vi "Beam_Max_Pos.vi"(0 "Beam Name":string, 1 "Traverse Name":string, 2 "Fixed Axis only?":bool, 5 "Fixed Axis":T1, 7 "Search Step (mm)":dbl=1.0, 9 "Starting Position":dbl[](array[numeric]) format="%.1f", 11 "Mode":T3, 12 "Wavelength  nm":sgl=533.0 caption="Wavelength (0.0)", 14 "Picture Log":path) -> (3 "Message":string, 4 "Beam maxima":dbl[](array[numeric]) format="%.1f", 10 "Status":T2, 15 "Power at Maxima":dbl)   [LabVIEW 2020]
uses:
  Controls/User_Specific_mode.ctl
  Gen Trav/Multi_Run_Status.ctl
  Controls/Fixed Axis.ctl
  Gen Trav/Trav_mode.ctl
  Controls/Tunnel_Coordinates.ctl
panel:
  out "vi reference":refnum<vi>
  in  "stop":bool
  out "Y":i32
  out "X":i32
  out "Array 2":dbl[](array[numeric]) format="%.4f"
  out "Measured Points":dbl[][](array[numeric]) format="%.2f"
  out "Current Value":dbl format="%.2f"
  out "Current Index":i32
  out "Array":i32[][](array[numeric])
  out "Light Power Measurement":dbl[][](graph)
  out "Found Maxima?":bool
  out "Present Position":dbl[](array[numeric])
  out "Profile":dbl[][](array[numeric]) format="%.2f"
  out "Log File":path
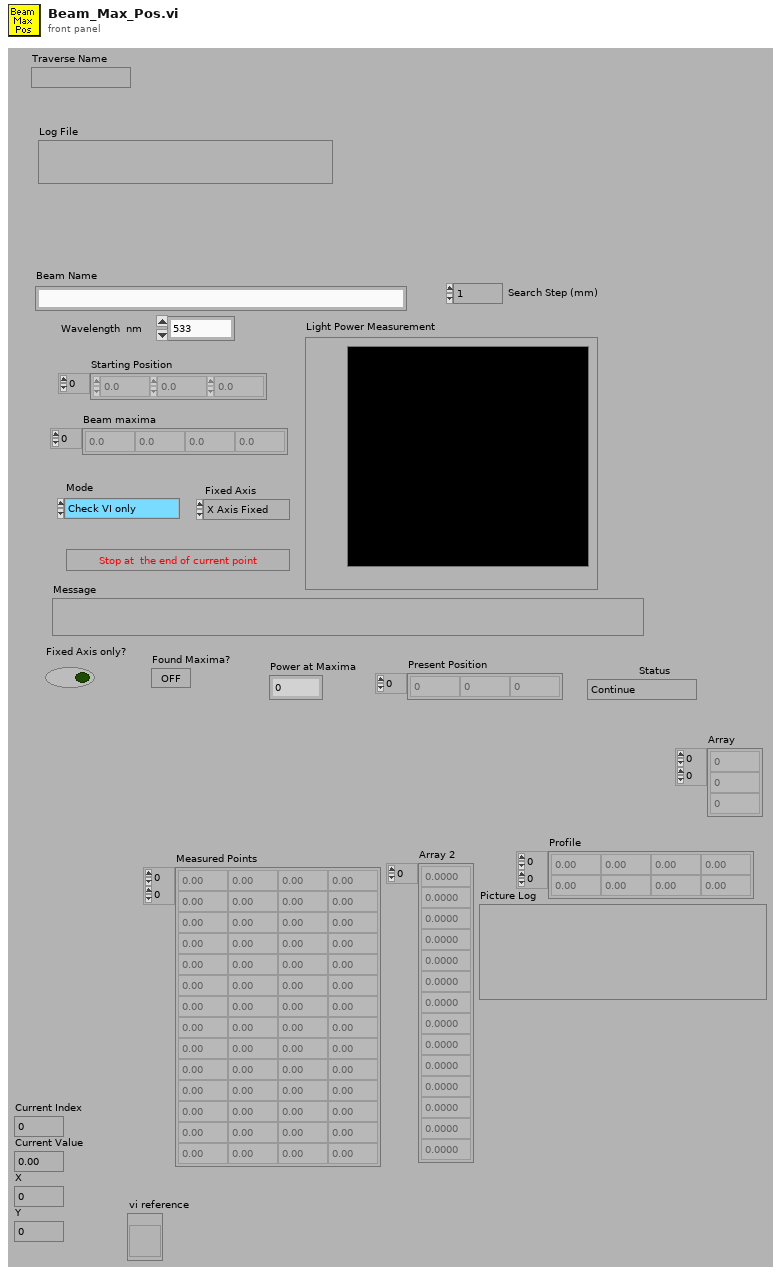
[diagram p1: front panel]
types:
  T1 = typedef "Fixed Axis.ctl" = enum16{"X Axis Fixed", "Y Axis Fixed", "Z Axis Fixed"}
  T2 = typedef "Multi_Run_Status.ctl" = enum16{"Continue", "Continue with Error", "Jump to Next Point", "Jump to Next Row", "Jump To Fall Back", "Terminate Run"}
  T3 = typedef "User_Specific_mode.ctl" = enum16{"Check VI only", "Run VI"}
  T4 = typedef "Tunnel_Coordinates.ctl" = enum16{"Work in Tunnel Coordinates", "Work in Model Coordinates"}
  T5 = typedef "Trav_mode.ctl" = enum16{"Move traverse", "Read traverse position", "Teach Position"}
  T6 = cluster{"second":i32, "minute":i32, "hour":i32, "day of month":i32, "month":i32, "year":i32, "day of week":i32, "day of year":i32, "is DST":i32}
  T7 = typedef "LVRectTypeDef.ctl" = cluster{"left":i16, "top":i16, "right":i16, "bottom":i16}
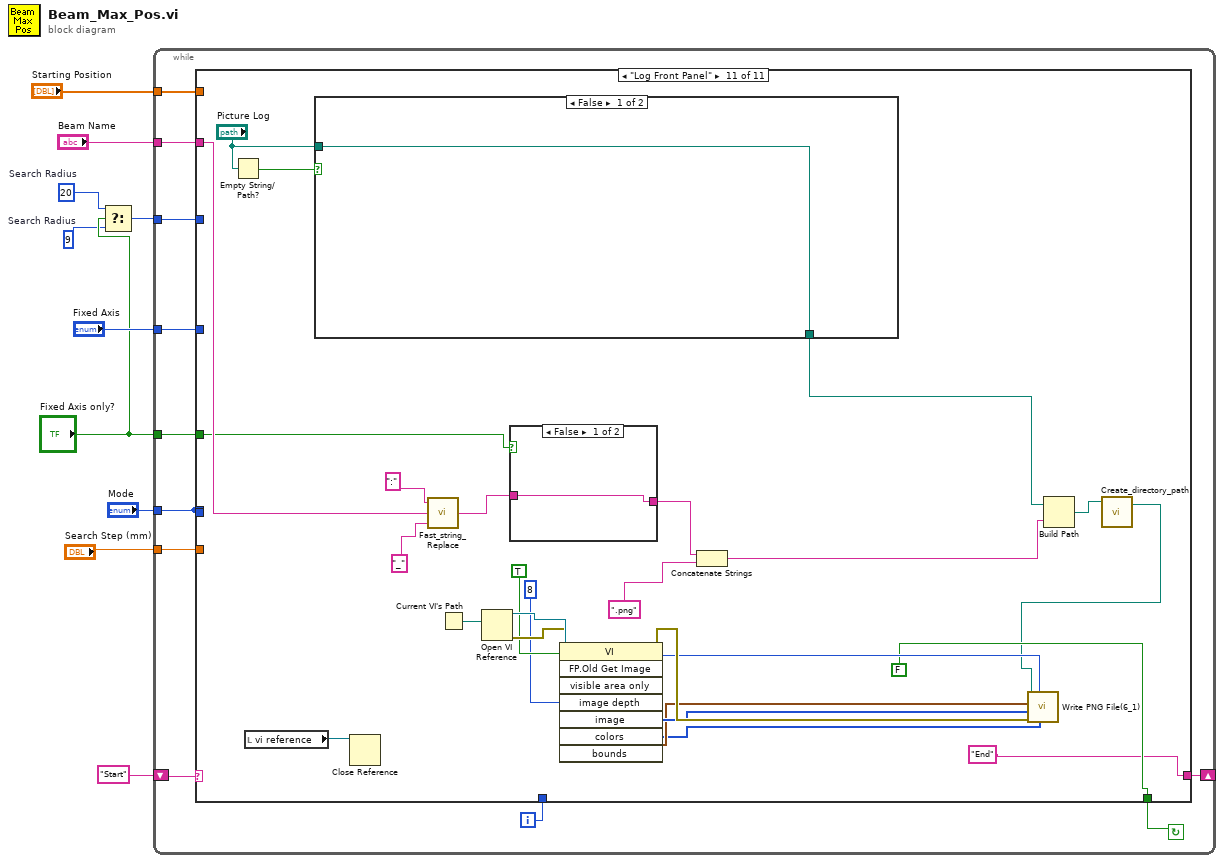
[diagram p0: block diagram]
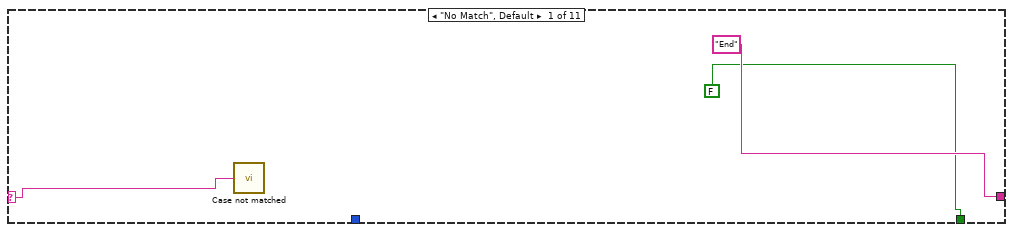
[diagram p2: hidden frame]
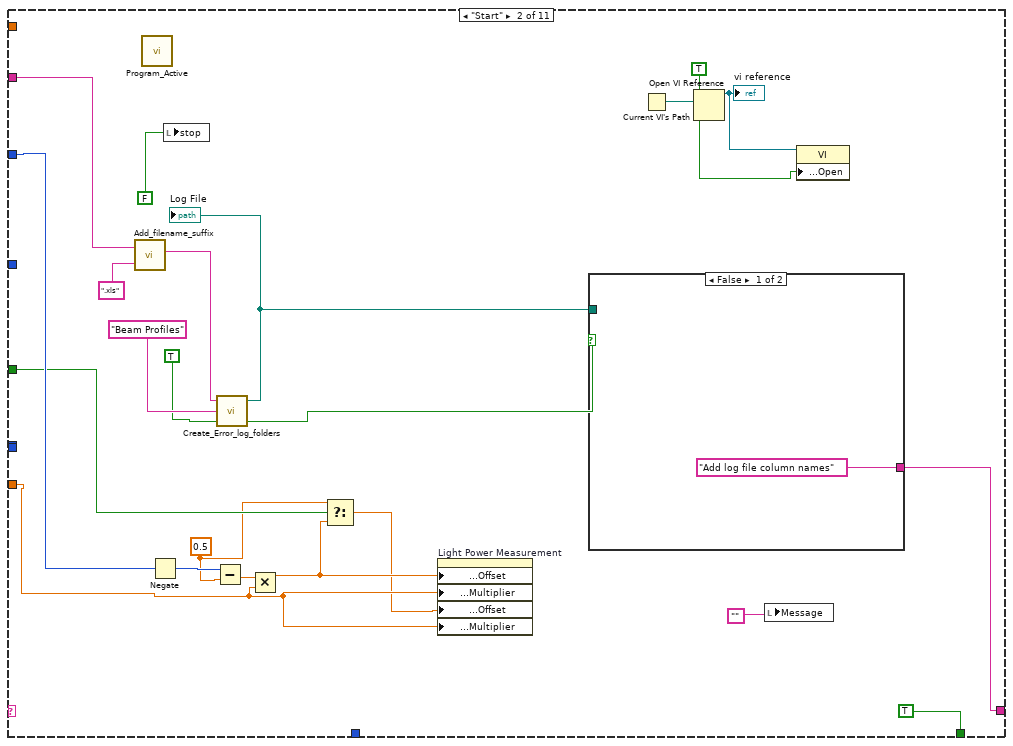
[diagram p3: hidden frame]
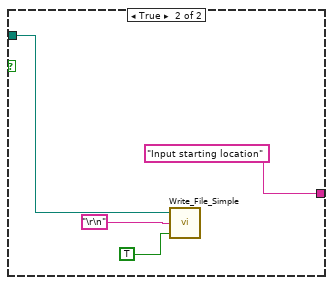
[diagram p4: hidden frame]
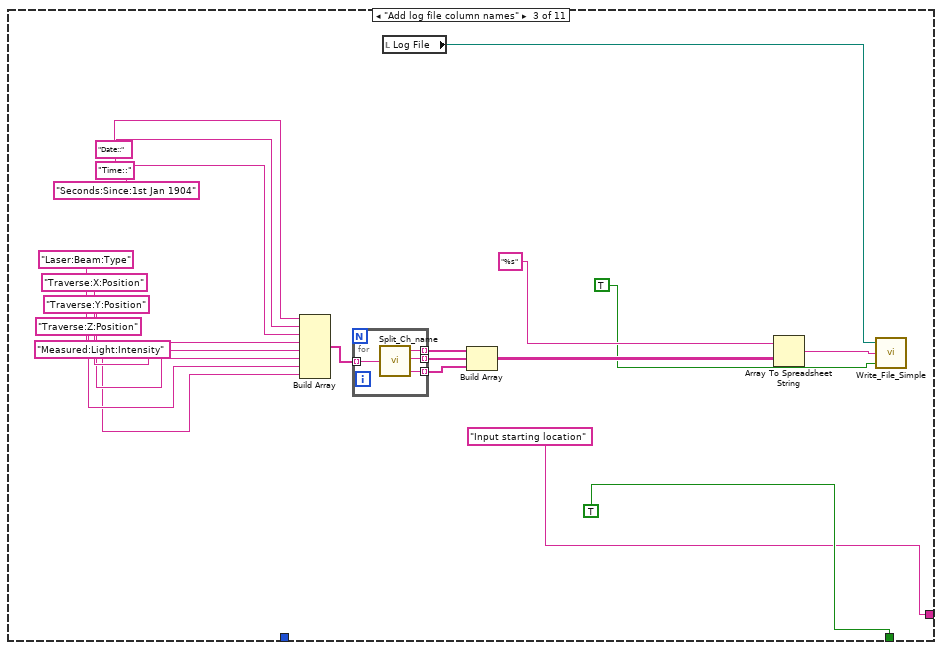
[diagram p5: hidden frame]
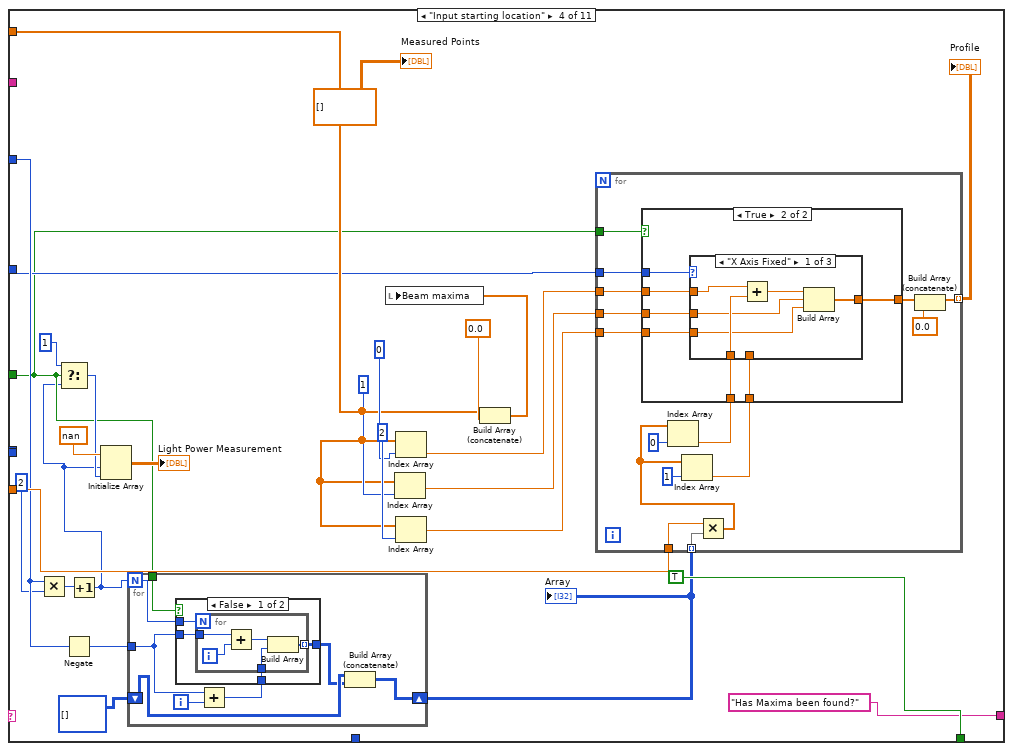
[diagram p6: hidden frame]
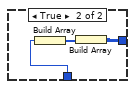
[diagram p7: hidden frame]
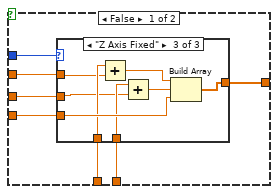
[diagram p8: hidden frame]
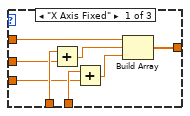
[diagram p9: hidden frame]
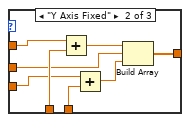
[diagram p10: hidden frame]
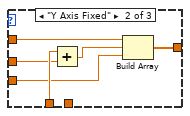
[diagram p11: hidden frame]
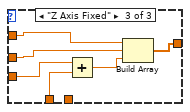
[diagram p12: hidden frame]
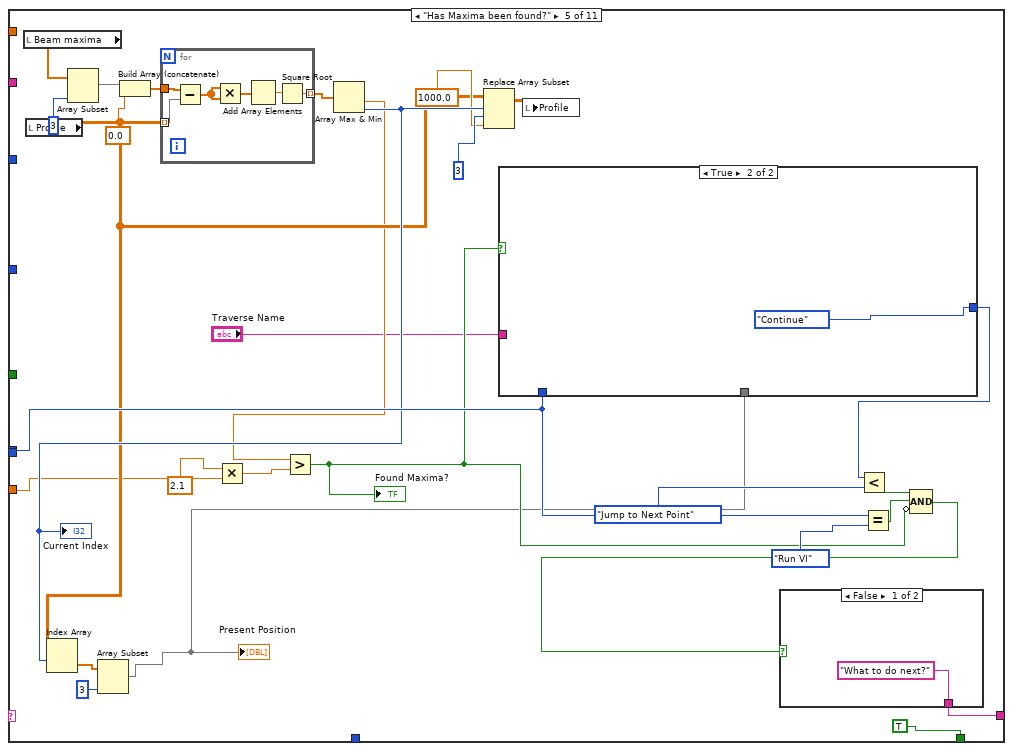
[diagram p13: hidden frame]
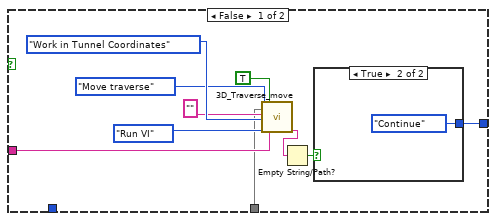
[diagram p14: hidden frame]
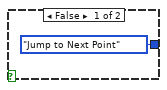
[diagram p15: hidden frame]
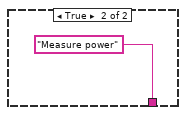
[diagram p16: hidden frame]
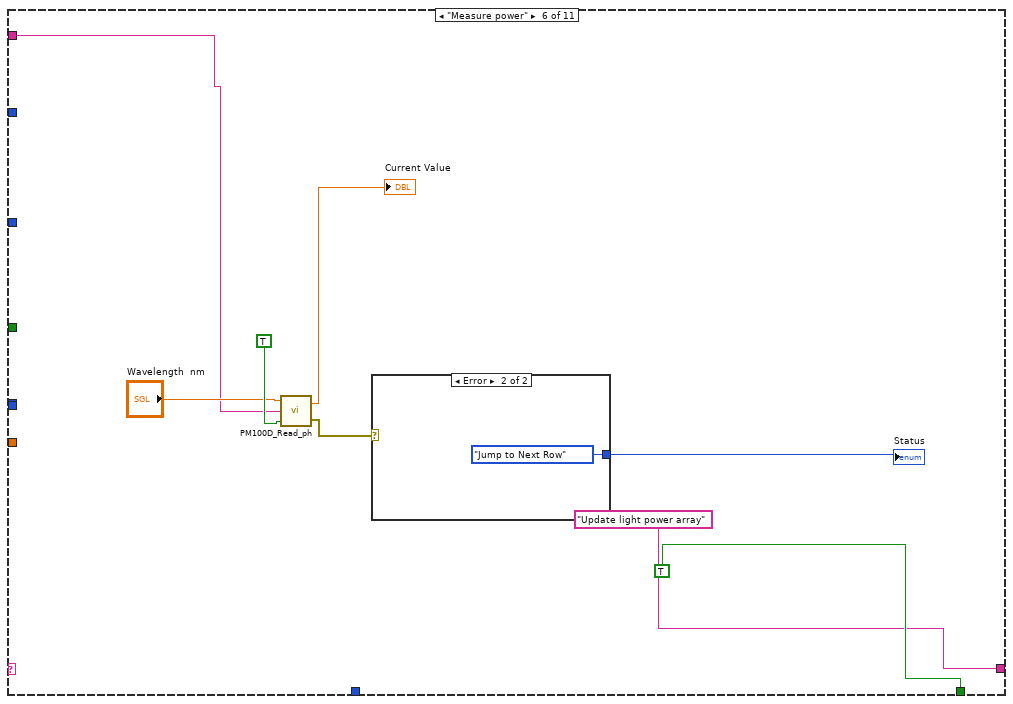
[diagram p17: hidden frame]
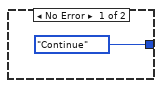
[diagram p18: hidden frame]
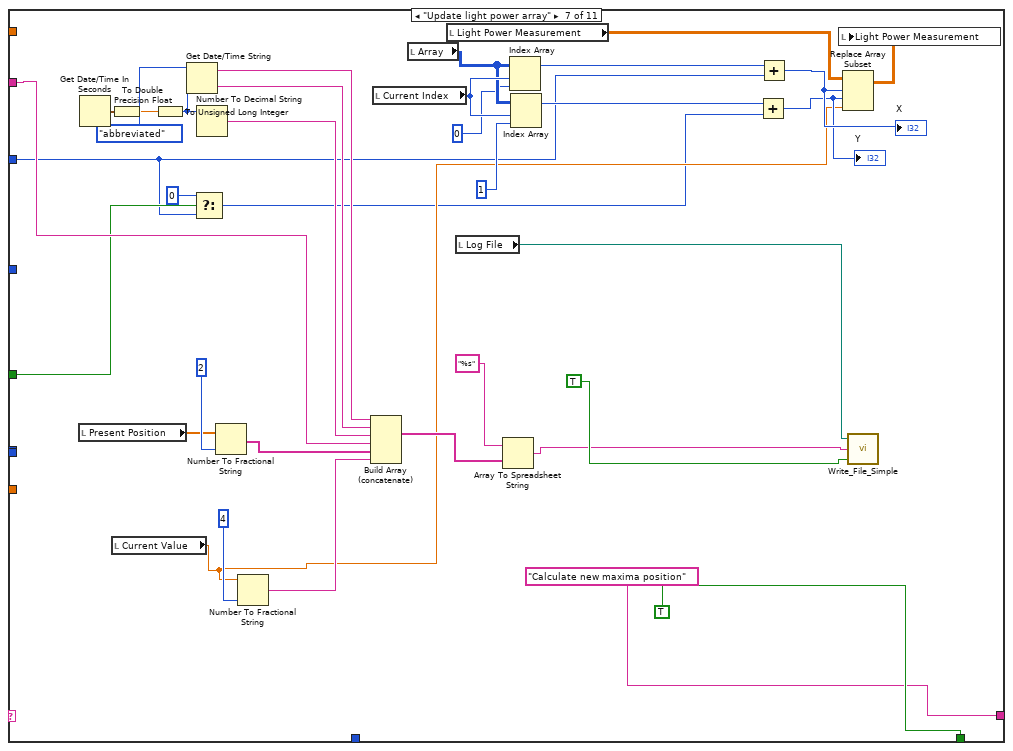
[diagram p19: hidden frame]
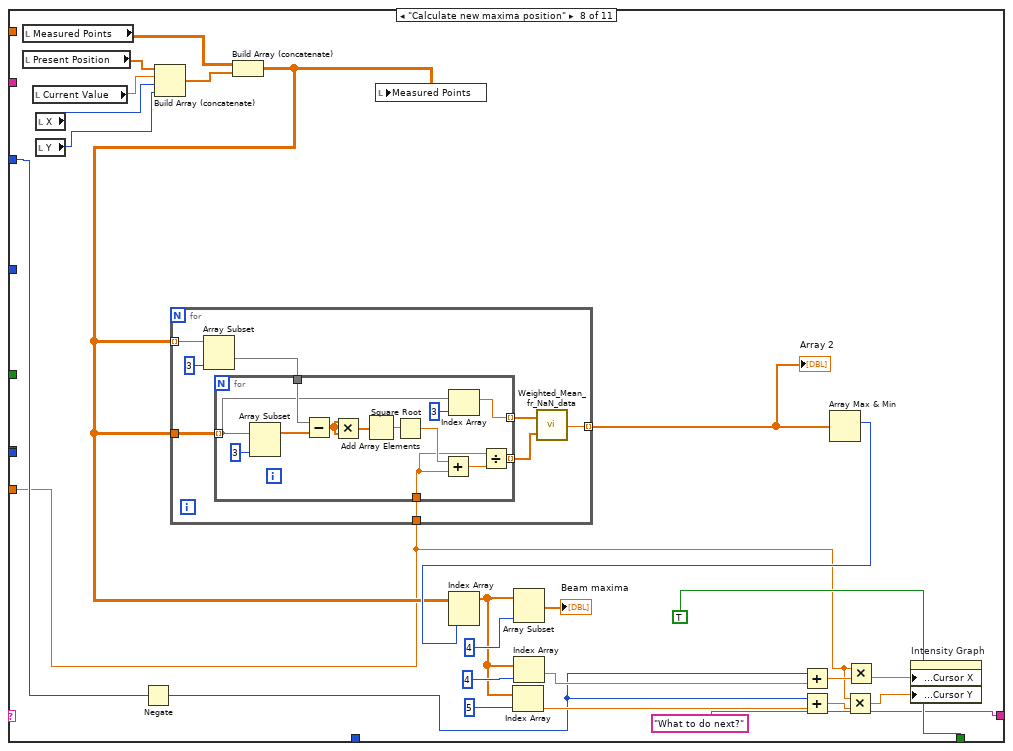
[diagram p20: hidden frame]
diagram:
  w1 = 20  # Search Radius
  w2 = 9  # Search Radius
  n1 = Select(t=w1, s="Fixed Axis only?", f=w2) -> (s? t:f=w4:i32)
  n2 = while {
    tunnel: "Search Step (mm)" -> [w18]
    tunnel: "Mode" -> [w19]
    shift-left: "Start" -> [w13]
    shift-right: [w20] -> _
    tunnel: w4 -> [w17]
    tunnel: "Beam Name" -> [w16]
    tunnel: "Starting Position" -> [w15]
    tunnel: "Fixed Axis" -> [w12]
    tunnel: "Fixed Axis only?" -> [w11]
    i -> [w14]
    stop <- w21 continue-if-true
    n3 = case shown="\"Log Front Panel\"" w13 {
      selector: w13 -> [w22 _ _ _ _ _ _ _ _ _ _]
      tunnel: w19 -> [_ _ _ _ w219 _ _ _ w340 _ _]
      tunnel: [FALSE TRUE TRUE TRUE TRUE TRUE TRUE TRUE w334 TRUE FALSE] -> w21
      tunnel: ["End" w36 "Input starting location" "Has Maxima been found?" w200 "Update light power array" "Calculate new maxima position" "What to do next?" w337 "Log Front Panel" "End"] -> w20
      tunnel: w19 -> [_ _ _ _ _ _ _ _ _ _ _]
      tunnel: w18 -> [_ w31 _ w94 w201 _ _ w291 _ _ _]
      tunnel: w17 -> [_ w41 _ w88 _ _ w255 w295 _ _ _]
      tunnel: w16 -> [_ w39 _ _ _ w243 w261 _ _ w358 w407]
      tunnel: w15 -> [_ _ _ w82 _ _ _ _ _ w357 _]
      tunnel: w14 -> [_ _ _ _ _ _ _ _ _ _ _]
      tunnel: w12 -> [_ _ _ w80 _ _ _ _ _ _ _]
      tunnel: w11 -> [_ w28 _ w76 _ _ w256 _ _ _ w404]
      frame "No Match", Default {
        n4 = call "Case not matched.vi"("Case Name not Matched"=w22) -> ()
      }
      frame "Start" {
        w25 = 0.5 ("y")
        n5 = call "Add_filename_suffix.vi"("Filename"=w39, "Suffix to add"=".xls") -> ("Filename out"=w37:string)  [unwired: 3 out]
        n6 = call "Program_Active.vi"() -> ()  [unwired: 1 in]
        n7 = Negate(x=w41) -> (-x=w29:i32)
        n8 = local write "stop"(FALSE ("stop")) -> ()
        n9 = Subtract(x=w29, y=w25) -> (x-y=w30:dbl)
        n10 = call "Create_Error_log_folders.vi"("Log Filename"=w37, "Log Folder"="Beam Profiles" ("Input Element"), "Per Day Log File?"=TRUE) -> ("Local Log File"=w45:path, "exists?"=w44:bool)  [unwired: 3 in]
        "Log File" <- w45
        n11 = Multiply(x=w30, y=w31) -> (x*y=w27:dbl)
        n12 = Select(t=w25, s=w28, f=w27) -> (s? t:f=w26:dbl)
        n13 = property on="Light Power Measurement" class="IntGraph (strict)"("X Scale.Offset and Multiplier:Offset"=w27, "X Scale.Offset and Multiplier:Multiplier"=w31, "Y Scale.Offset and Multiplier:Offset"=w26, "Y Scale.Offset and Multiplier:Multiplier"=w31) -> ()  [unwired: 2 in, 2 out]
        n14 = case shown="False" w44 {
          tunnel: w45 -> [_ w48]
          tunnel: ["Add log file column names" "Input starting location"] -> w36
          frame False {
          }
          frame True {
            n15 = call "Write_File_Simple.vi"("append to file? (new file:F)"=TRUE, "character string"="\r\n", "file path"=w48) -> ()  [unwired: 2 out]
          }
        }
        n16 = Current VI's Path() -> (path=w35:path)
        n17 = Open VI Reference(vi path=w35) -> (vi reference=w34:refnum<vi>)  [unwired: 1 in, 5 out]
        "vi reference" <- w34
        n18 = local write "Message"("") -> ()
        n19 = property class="VI"(reference=w34, "Front Panel Window:Open"=TRUE) -> ()  [unwired: 1 in, 2 out]
      }
      frame "Add log file column names" {
        n20 = Build Array("Date::", "Time::", "Seconds:Since:1st Jan 1904", "Laser:Beam:Type", "Traverse:X:Position", "Traverse:Y:Position", "Traverse:Z:Position", "Measured:Light:Intensity") -> (w64:string[])
        n21 = for {
          tunnel: w64 -> [w74] mode=indexing
          tunnel: [w73] -> w65 mode=indexing
          tunnel: [w72] -> w66 mode=indexing
          tunnel: [w71] -> w67 mode=indexing
          n22 = call "Split_Ch_name.vi"("Ch name"=w74) -> ("Top level"=w73:string, "Middle"=w72:string, "Low level"=w71:string)
        }
        n23 = local read "Log File"() -> (w52:path)
        n24 = Build Array(w65, w66, w67) -> (w62:string[][])
        n25 = Array To Spreadsheet String(array=w62, 3:"%s" ("format string")) -> (spreadsheet string=w53:string)  [unwired: 1 out]
        n26 = call "Write_File_Simple.vi"("append to file? (new file:F)"=TRUE, "character string"=w53, "file path"=w52) -> ()  [unwired: 2 out]
      }
      frame "Input starting location" {
        n27 = Multiply(x=w88, y=2) -> (x*y=w86:i32)
        n28 = Negate(x=w88) -> (-x=w77:i32)
        n29 = Increment(x=w86) -> (x+1=w75:i32)
        n30 = Select(t=1, s=w76, f=w75) -> (s? t:f=w78:i32)
        n31 = Initialize Array(nan, w75, w78) -> (→"Light Power Measurement":dbl[][])
        n32 = for {
          N: w75 -> [w102]
          tunnel: w77 -> [w103]
          shift-right: [w105] -> w92
          shift-left: i32[][] [] -> [w107]
          tunnel: w76 -> [w104]
          i -> [w109]
          n33 = Add(x=w103, y=w109) -> (x+y=w108:i32)
          n34 = case shown="False" w104 {
            tunnel: w108 -> [w113 w120]
            tunnel: [w112 w121] -> w106
            tunnel: w103 -> [w111 _]
            tunnel: w102 -> [w110 _]
            frame False {
              n35 = for {
                N: w110 -> [_]
                tunnel: w111 -> [w117]
                tunnel: w113 -> [w115]
                tunnel: [w114] -> w112 mode=indexing
                i -> [w118]
                n36 = Add(x=w117, y=w118) -> (x+y=w116:i32)
                n37 = Build Array(w116, w115) -> (w114:i32[])
              }
            }
            frame True {
              n38 = Build Array(w120) -> (w119:i32[])
              n39 = Build Array(w119) -> (w121:i32[][])
            }
          }
          n40 = Build Array (concatenate)(w107, w106) -> (w105:i32[][])
        }
        "Array" <- w92
        n41 = Index Array(array=w82, index=1 ("Index")) -> (element=w98:dbl)
        n42 = Index Array(array=w82, index=0 ("Index")) -> (element=w99:dbl)
        n43 = Index Array(array=w82, index=2 ("Index")) -> (element=w97:dbl)
        n44 = Build Array (concatenate)(w82, 0.0 ("Numeric")) -> (w95:dbl[])
        n45 = local write "Beam maxima"(w95) -> ()
        n46 = for {
          tunnel: w94 -> [w136]
          tunnel: w92 -> [w135] mode=indexing
          tunnel: w80 -> [w134]
          tunnel: w99 -> [w130]
          tunnel: w98 -> [w127]
          tunnel: w97 -> [w126]
          tunnel: [w124] -> w100 mode=indexing
          tunnel: w76 -> [w122]
          n47 = Multiply(x=w136, y=w135) -> (x*y=w131:dbl[])
          n48 = Index Array(array=w131, index=0 ("Index")) -> (element=w129:dbl)
          n49 = Index Array(array=w131, index=1 ("Index")) -> (element=w128:dbl)
          n50 = case shown="True" w122 {
            tunnel: w134 -> [w143 w174]
            tunnel: w130 -> [w142 w173]
            tunnel: w129 -> [w141 w172]
            tunnel: w128 -> [w140 w171]
            tunnel: w127 -> [w139 w170]
            tunnel: w126 -> [w138 w169]
            tunnel: [w137 w168] -> w125
            frame False {
              n51 = case shown="\"Z Axis Fixed\"" w143 {
                tunnel: w142 -> [w151 w158 w162]
                tunnel: w141 -> [w150 w156 w165]
                tunnel: w140 -> [w149 w155 w164]
                tunnel: w139 -> [w148 w152 w163]
                tunnel: w138 -> [w147 w154 w166]
                tunnel: [w144 w159 w167] -> w137
                frame "X Axis Fixed" {
                  n52 = Add(x=w150, y=w148) -> (x+y=w146:dbl)
                  n53 = Add(x=w149, y=w147) -> (x+y=w145:dbl)
                  n54 = Build Array(w151, w146, w145) -> (w144:dbl[])
                }
                frame "Y Axis Fixed" {
                  n55 = Add(x=w158, y=w156) -> (x+y=w157:dbl)
                  n56 = Add(x=w154, y=w155) -> (x+y=w153:dbl)
                  n57 = Build Array(w157, w152, w153) -> (w159:dbl[])
                }
                frame "Z Axis Fixed" {
                  n58 = Add(x=w165, y=w162) -> (x+y=w161:dbl)
                  n59 = Add(x=w164, y=w163) -> (x+y=w160:dbl)
                  n60 = Build Array(w161, w160, w166) -> (w167:dbl[])
                }
              }
            }
            frame True {
              n61 = case shown="\"X Axis Fixed\"" w174 {
                tunnel: w173 -> [w179 w186 w191]
                tunnel: w172 -> [w177 w185 w188]
                tunnel: w171 -> [_ _ _]
                tunnel: w170 -> [w176 w184 w190]
                tunnel: w169 -> [w175 w181 w189]
                tunnel: [w180 w182 w192] -> w168
                frame "X Axis Fixed" {
                  n62 = Add(x=w179, y=w177) -> (x+y=w178:dbl)
                  n63 = Build Array(w178, w176, w175) -> (w180:dbl[])
                }
                frame "Y Axis Fixed" {
                  n64 = Add(x=w185, y=w184) -> (x+y=w183:dbl)
                  n65 = Build Array(w186, w183, w181) -> (w182:dbl[])
                }
                frame "Z Axis Fixed" {
                  n66 = Add(x=w189, y=w188) -> (x+y=w187:dbl)
                  n67 = Build Array(w191, w190, w187) -> (w192:dbl[])
                }
              }
            }
          }
          n68 = Build Array (concatenate)(w125, 0.0 ("Input Element")) -> (w124:dbl[])
        }
        "Profile" <- w100
        "Measured Points" <- dbl[][] [] ("Measured Points")
      }
      frame "Has Maxima been found?" {
        n69 = local read "Beam maxima"() -> (w217:dbl[])
        n70 = local read "Profile"() -> (w207:dbl[][])
        n71 = Array Subset(array=w217, length=3 ("Array Length")) -> (w214:dbl[])  [unwired: 1 in]
        n72 = Build Array (concatenate)(w214, 0.0 ("Input Element")) -> (w213:dbl[])
        n73 = for {
          tunnel: w207 -> [w242] mode=indexing
          tunnel: w213 -> [w241]
          tunnel: [w237] -> w215 mode=indexing
          n74 = Subtract(x=w241, y=w242) -> (x-y=w239:dbl[])
          n75 = Multiply(x=w239, y=w239) -> (x*y=w238:dbl[])
          n76 = Add Array Elements(numeric array=w238) -> (sum=w240:dbl)
          n77 = Square Root(x=w240) -> (sqrt(x)=w237:dbl)
        }
        n78 = Multiply(x=2.1, y=w201) -> (x*y=w204:dbl)
        n79 = Array Max & Min(array=w215) -> (min value=w205:dbl, min index (indices)=w211:i32)  [unwired: 2 out]
        "Current Index" <- w211
        n80 = Index Array(array=w207, index (row)=w211) -> (element=w197:dbl[])  [unwired: 1 in]
        n81 = Array Subset(array=w197, length=3) -> (w194:dbl[])  [unwired: 1 in]
        "Present Position" <- w194
        n82 = Greater?(x=w205, y=w204) -> (0:w198:bool)
        "Found Maxima?" <- w198
        n83 = Replace Array Subset(array=w207, new element=1000.0 ("Element Data"), index (row)=w211, index (col)=3 ("Index")) -> (w208:dbl[][])
        n84 = case shown="True" w198 {
          tunnel: w219 -> [_ _]
          tunnel: "Traverse Name" -> [w226 _]
          tunnel: w194 -> [w225 _]
          tunnel: [w222 Multi_Run_Status."Continue" ("Status")] -> w193
          frame False {
            n85 = call "3D_Traverse_move.vi"("Mode"=Trav_mode."Move traverse", "Position"=w225, "Extra command String"="", "Work in Tunnel Coordinates"=Tunnel_Coordinates."Work in Tunnel Coordinates", "Simulate/Run"=User_Specific_mode."Run VI", "Route Checking?"=TRUE, "Traverse name"=w226) -> ("Error String"=w224:string)  [unwired: 9 in, 3 out]
            n86 = Empty String/Path?(string/path=w224) -> (empty?=w223:bool)
            n87 = case shown="True" w223 {
              tunnel: [Multi_Run_Status."Jump to Next Point" ("Status") Multi_Run_Status."Continue" ("Status")] -> w222
              frame False {
              }
              frame True {
              }
            }
          }
          frame True {
          }
        }
        n88 = local write "Profile"(w208) -> ()
        n89 = Less?(x=w193, y=Multi_Run_Status."Jump to Next Point" ("Status")) -> (x < y?=w203:bool)
        n90 = Equal?(x=w219, y=User_Specific_mode."Run VI" ("Mode")) -> (x = y?=w202:bool)
        n91 = Compound Arithmetic op=AND(w203, w202, invert w198) -> (w199:bool)
        n92 = case shown="False" w199 {
          tunnel: ["What to do next?" "Measure power"] -> w200
          frame False {
          }
          frame True {
          }
        }
      }
      frame "Measure power" {
        n93 = call "PM100D_Read_ph.vi"("stop"=TRUE, "Beam Name"=w243, "Wavelength (0.0)"="Wavelength  nm") -> ("error out"=w245:errorcluster, "Average Power (mW)"=→"Current Value":dbl)
        n94 = case shown="Error" w245 {
          tunnel: [Multi_Run_Status."Continue" ("Status") Multi_Run_Status."Jump to Next Row" ("Status")] -> w244
          frame No Error {
          }
          frame Error {
          }
        }
        "Status" <- w244
      }
      frame "Update light power array" {
        n95 = local read "Present Position"() -> (w274:dbl[])
        n96 = Get Date/Time In Seconds() -> (seconds since 1Jan1904=w263:timestamp)
        n97 = To Double Precision Float(number=w263) -> (double precision float=w284:dbl)
        n98 = local read "Current Value"() -> (w257:dbl)
        n99 = To Unsigned Long Integer(number=w284) -> (unsigned 32bit integer=w283:u32)
        n100 = Get Date/Time String(date format (0)=enum16{"short", "long", "abbreviated"}."abbreviated", seconds (now)=w283) -> (date string=w282:string, time string=w281:string)  [unwired: 1 out]
        n101 = Select(t=0, s=w256, f=w255) -> (s? t:f=w253:i32)
        n102 = Number To Decimal String(number=w283) -> (decimal integer string=w280:string)  [unwired: 1 out]
        n103 = Number To Fractional String(number=w274, precision (6)=i16 2) -> (F-format string=w275:string[])  [unwired: 2 out]
        n104 = Number To Fractional String(number=w257, precision (6)=i16 4) -> (F-format string=w276:string)  [unwired: 2 out]
        n105 = Build Array (concatenate)(w282, w281, w280, w261, w275, w276) -> (w279:string[])
        n106 = local read "Current Index"() -> (w273:i32)
        n107 = local read "Array"() -> (w272:i32[][])
        n108 = local read "Light Power Measurement"() -> (w269:dbl[][])
        n109 = local read "Log File"() -> (w258:path)
        n110 = Array To Spreadsheet String(array=w279, 3:"%s" ("format string")) -> (spreadsheet string=w259:string)  [unwired: 1 out]
        n111 = Index Array(array=w272, index (row)=w273, index (col)=0 ("Index")) -> (element=w266:i32)
        n112 = Index Array(array=w272, index (row)=w273, index (col)=1 ("Index")) -> (element=w267:i32)
        n113 = Add(x=w267, y=w253) -> (x+y=w264:i32)
        "Y" <- w264
        n114 = Add(x=w266, y=w255) -> (x+y=w265:i32)
        "X" <- w265
        n115 = Replace Array Subset(array=w269, new element=w257, index (row)=w265, index (col)=w264) -> (w268:dbl[][])
        n116 = local write "Light Power Measurement"(w268) -> ()
        n117 = call "Write_File_Simple.vi"("append to file? (new file:F)"=TRUE, "character string"=w259, "file path"=w258) -> ()  [unwired: 2 out]
      }
      frame "Calculate new maxima position" {
        n118 = local read "Measured Points"() -> (w311:dbl[][])
        n119 = local read "Present Position"() -> (w310:dbl[])
        n120 = local read "Current Value"() -> (w309:dbl)
        n121 = local read "X"() -> (w304:i32)
        n122 = local read "Y"() -> (w303:i32)
        n123 = Negate(x=w295) -> (-x=w293:i32)
        n124 = Build Array (concatenate)(w310, w309, w304, w303) -> (w308:dbl[])
        n125 = Build Array (concatenate)(w311, w308) -> (w305:dbl[][])
        n126 = for {
          tunnel: w305 -> [w320] mode=indexing
          tunnel: w305 -> [w318]
          tunnel: w291 -> [w316]
          tunnel: [w313] -> w307 mode=indexing
          n127 = Array Subset(array=w320, length=3 ("Array Length")) -> (w317:dbl[])  [unwired: 1 in]
          n128 = for {
            tunnel: w318 -> [w327] mode=indexing
            tunnel: w317 -> [w332]
            tunnel: w316 -> [w322]
            tunnel: [w324] -> w314 mode=indexing
            tunnel: [w321] -> w315 mode=indexing
            n129 = Array Subset(array=w327, length=3 ("Array Length")) -> (w331:dbl[])  [unwired: 1 in]
            n130 = Subtract(x=w332, y=w331) -> (x-y=w328:dbl[])
            n131 = Multiply(x=w328, y=w328) -> (x*y=w329:dbl[])
            n132 = Add Array Elements(numeric array=w329) -> (sum=w330:dbl)
            n133 = Square Root(x=w330) -> (sqrt(x)=w325:dbl)
            n134 = Add(x=w325, y=w322) -> (x+y=w323:dbl)
            n135 = Index Array(array=w327, index=3 ("Index")) -> (element=w321:dbl)
            n136 = Divide(x=w322, y=w323) -> (x/y=w324:dbl)
          }
          n137 = call "Weighted_Mean_fr_NaN_data.vi"("Weighting"=w314, "Data"=w315) -> ("Mean value"=w313:dbl)
        }
        "Array 2" <- w307
        n138 = local write "Measured Points"(w305) -> ()
        n139 = Array Max & Min(array=w307) -> (max index (indices)=w306:i32)  [unwired: 3 out]
        n140 = Index Array(array=w305, index (row)=w306) -> (element=w298:dbl[])  [unwired: 1 in]
        n141 = Index Array(array=w298, index=5 ("Index")) -> (element=w296:dbl)
        n142 = Array Subset(array=w298, length=4 ("Array Length")) -> (→"Beam maxima":dbl[])  [unwired: 1 in]
        n143 = Index Array(array=w298, index=4 ("Index")) -> (element=w297:dbl)
        n144 = Add(x=w293, y=w297) -> (x+y=w292:dbl)
        n145 = Add(x=w293, y=w296) -> (x+y=w290:dbl)
        n146 = Multiply(x=w291, y=w290) -> (x*y=w289:dbl)
        n147 = Multiply(x=w291, y=w292) -> (x*y=w288:dbl)
        n148 = property on="Intensity Graph" class="IntGraph (strict)"("Cursor.Cursor Position:Cursor X"=w288, "Cursor.Cursor Position:Cursor Y"=w289) -> ()  [unwired: 2 in, 2 out]
      }
      frame "What to do next?" {
        n149 = local read "Found Maxima?"() -> (w342:bool)
        n150 = case shown="False" "stop" {
          tunnel: [w344 w345] -> w338
          frame False {
            n151 = local read "Status"() -> (w344:T2)
          }
          frame True {
            w345 = Multi_Run_Status."Terminate Run" ("Status")
            n152 = local write "Status"(w345) -> ()
          }
        }
        n153 = case shown="False" w342 {
          tunnel: ["Has Maxima been found?" "Compile Message"] -> w337
          frame False {
          }
          frame True {
          }
        }
        n154 = Equal?(x=w340, y=User_Specific_mode."Run VI" ("Mode")) -> (x = y?=w336:bool)
        n155 = Less?(x=w338, y=Multi_Run_Status."Jump to Next Point" ("Status")) -> (x < y?=w335:bool)
        n156 = And(x=w335, y=w336) -> (x .and. y?=w334:bool)
      }
      frame "Compile Message" {
        # "X Y Z Power"
        n157 = local read "Beam maxima"() -> (w356:dbl[])
        n158 = Build Array("X", "Y", "Z", "Power" ("Input Element")) -> (w363:string[])
        n159 = Index Array(array=w356, index=3) -> (element=w354:dbl)
        n160 = for {
          tunnel: w356 -> [w380] mode=indexing
          shift-right: [w378] -> w362
          shift-left: "" -> [w379]
          tunnel: w363 -> [w377] mode=indexing
          tunnel: [w376] -> w359 mode=indexing
          tunnel: w357 -> [w375]
          i -> [w374]
          n161 = case shown="0, Default" w374 {
            tunnel: w380 -> [w381 w399]
            tunnel: w379 -> [w389 w397]
            tunnel: [w388 w396] -> w378
            tunnel: w377 -> [w382 w401]
            tunnel: [w386 TRUE] -> w376
            tunnel: w375 -> [w385 _]
            tunnel: w374 -> [w384 _]
            frame 0, Default {
              n162 = Index Array(array=w385, index=w384) -> (element=w383:dbl)
              n163 = Subtract(x=w381, y=w383) -> (x-y=w387:dbl)
              n164 = Equal To 0?(x=w387) -> (x = 0?=w386:bool)
              n165 = case shown="False" w386 {
                tunnel: w389 -> [w394 w395]
                tunnel: [w393 w395] -> w388
                tunnel: w382 -> [w392 _]
                tunnel: w387 -> [w390 _]
                frame False {
                  n166 = Format Into String(format string="%s=%.1fmm, " ("Format String"), initial string=w394, w392, w390) -> (resulting string=w393:string)  [unwired: 1 in, 1 out]
                }
                frame True {
                }
              }
            }
            frame 3 {
              n167 = Format Into String(format string="%s=%.1fmW" ("Format String"), initial string=w397, w401, w399) -> (resulting string=w396:string)  [unwired: 1 in, 1 out]
            }
          }
        }
        n168 = call "Orb_Calibration.vi"("Voltage"=w354) -> ("Normalised Voltage"=→"Power at Maxima":dbl)  [unwired: 1 out]
        n169 = And Array Elements(Boolean array=w359) -> (logical AND=w351:bool)
        n170 = case shown="False" w351 {
          tunnel: [w369 w372] -> w361
          tunnel: w358 -> [w368 w371]
          frame True {
            n171 = Format Into String(format string="%s position Unchanged " ("Format String"), w368) -> (resulting string=w369:string)  [unwired: 2 in, 1 out]
          }
          frame False {
            n172 = Format Into String(format string="%s position tweaked by " ("Format String"), w371) -> (resulting string=w372:string)  [unwired: 2 in, 1 out]
          }
        }
        n173 = Concatenate Strings(w361, w362, "\r\n") -> (→"Message":string)
      }
      frame "Log Front Panel" {
        w418 = 8 ("image depth")
        n174 = Empty String/Path?(string/path="Picture Log") -> (empty?=w416:bool)
        n175 = local read "vi reference"() -> (w410:refnum<vi>)
        n176 = case shown="False" w416 {
          tunnel: [w431 w434] -> w415
          tunnel: "Picture Log" -> [w431 _]
          frame False {
          }
          frame True {
            n177 = Get Date/Time In Seconds() -> (seconds since 1Jan1904=w433:timestamp)
            n178 = call <vilib>:"LV70TimeStampToDateRec.vi"("time stamp"=w433) -> ("date time rec"=w437:T6)
            n179 = Unbundle By Name(w437) -> ("day of month"=w440:i32, "hour"=w439:i32, "minute"=w438:i32)
            n180 = call "Create_Error_log_folders.vi"("Log Filename"="test", "Log Folder"="Beam_Max_Pos" ("name or relative path")) -> ("Local Log File"=w432:path)  [unwired: 4 in, 1 out]
            n181 = Strip Path(path=w432) -> (stripped path=w436:path)  [unwired: 1 out]
            n182 = Format Into String(format string="Day%02d_Time%02d-%02d", w440, w439, w438) -> (resulting string=w435:string)  [unwired: 2 in, 1 out]
            n183 = Build Path(base path=w436, name or relative path=w435) -> (appended path=w434:path)
          }
        }
        n184 = Close Reference(reference=w410) -> ()  [unwired: 1 in, 1 out]
        n185 = call "Fast_string_Replace.vi"("Replace match with:"="_", "Input String"=w407, "regular expression"=":") -> ("Output String"=w403:string)  [unwired: 1 in, 1 out]
        n186 = Current VI's Path() -> (path=w426:path)
        n187 = Open VI Reference(vi path=w426) -> (vi reference=w425:refnum<vi>, error out=w424:errorcluster)  [unwired: 1 in, 4 out]
        n188 = case shown="False" w404 {
          tunnel: w403 -> [w427 w430]
          tunnel: [w427 w429] -> w402
          frame False {
          }
          frame True {
            n189 = Concatenate Strings(w430, "_1D" ("string")) -> (w429:string)
          }
        }
        n190 = invoke class="VI" method="FP.Old Get Image"(reference=w425, error in=w424, "visible area only"=TRUE, "image depth"=w418) -> (error out=w422:errorcluster, "image"=w421:u8[], "colors"=w419:u32[], "bounds"=w420:T7)  [unwired: 4 in, 4 out]
        n191 = Concatenate Strings(w402, ".png" ("string")) -> (w412:string)
        n192 = Build Path(base path=w415, name or relative path=w412) -> (appended path=w409:path)
        n193 = call "Create_directory_path.vi"("Path name"=w409) -> ("Path name Out"=w408:path)  [unwired: 2 in, 1 out]
        n194 = call <vilib>:"Write PNG File(6_1).vi"("color table"=w419, "depth"=w418, "error in (no error)"=w422, "flattened image data"=w421, "rect"=w420, "path to PNG file"=w408) -> ()  [unwired: 6 out]
      }
    }
  }
